vi "Post-Build Action.vi"(5 "Files Generated by Build":path[](array[path]), 6 "Top Level/Always Included VIs":path[](array[path]), 7 "Destination Path":path, 8 "error in (no error)":errorcluster, 9 "Target Name":string, 10 "Build Specification Name":string, 11 "Project Path":path) -> (0 "error out":errorcluster)   [LabVIEW 2023]
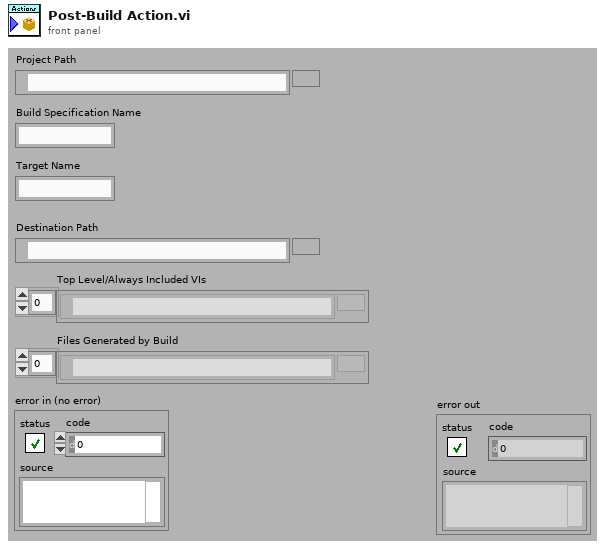
[diagram p1: front panel]
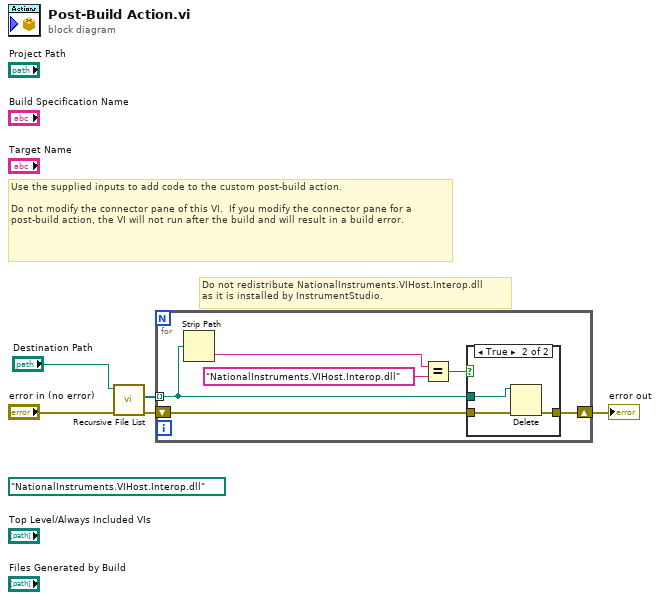
[diagram p0: block diagram]
diagram:
  (unwired) path "NationalInstruments.VIHost.Interop.dll" ("name or relative path")
  # "Do not redistribute NationalInstruments.VIHost.Interop.dll \nas it is installed by InstrumentStudio."
  # "Use the supplied inputs to add code to the custom post-build action.\n\nDo not modify the connector pane of this VI.  If you modify the connector pane for a post-build action, the VI will not run after the build and will result in a build error."
  n1 = call <vilib>:"Recursive File List.vi"("error in (no error)"="error in (no error)", "Folder Path"="Destination Path") -> ("error out"=w2:errorcluster, "All Files in Dir"=w3:path[])  [unwired: 5 in, 3 out]
  n2 = for {
    tunnel: w3 -> [w8] mode=indexing
    shift-right: [w6] -> w1
    shift-left: w2 -> [w7]
    n3 = Strip Path(path=w8) -> (name=w11:string)  [unwired: 1 out]
    n4 = Equal?(x=w11, y="NationalInstruments.VIHost.Interop.dll") -> (x = y?=w9:bool)
    n5 = case shown="True" w9 {
      tunnel: w8 -> [_ w15]
      tunnel: w7 -> [w12 w14]
      tunnel: [w12 w13] -> w6
      frame False {
      }
      frame True {
        n6 = Delete(path (use dialog)=w15, error in=w14) -> (error out=w13:errorcluster)  [unwired: 3 in, 2 out]
      }
    }
  }
  "error out" <- w1
